vi "Inc_Dec_Builder.vi"(8 "error in (no error)":errorcluster, 9 "Index_Str_In":string, 10 "Array In":i32[](array[numeric])) -> (0 "error out":errorcluster, 2 "Array":i32[](array[numeric]))   [LabVIEW 2017]
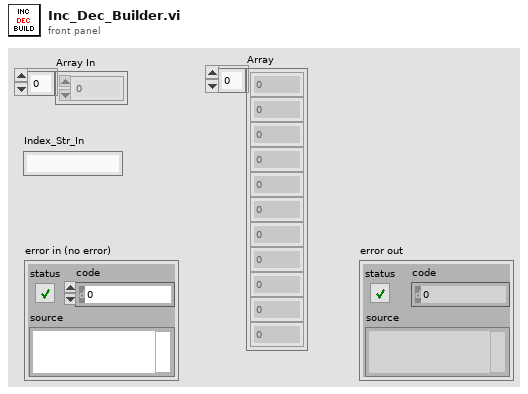
[diagram p1: front panel]
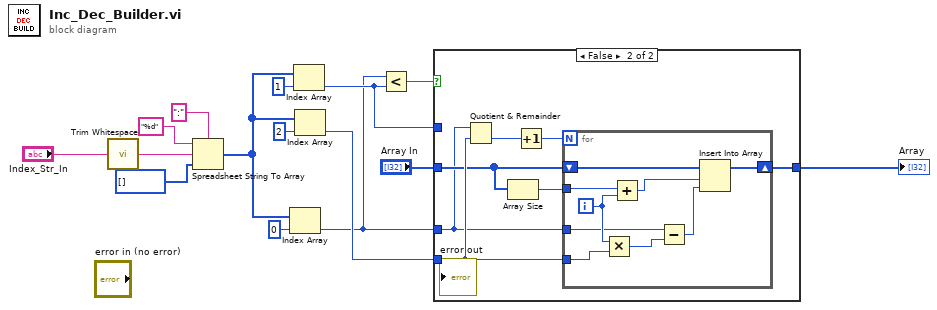
[diagram p0: block diagram]
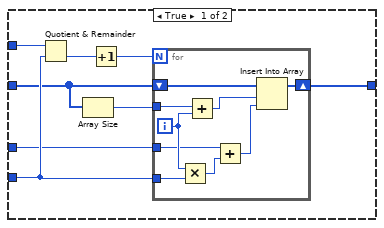
[diagram p2: hidden frame]
diagram:
  n1 = call <vilib>:"Trim Whitespace.vi"("string"="Index_Str_In") -> ("trimmed string"=w13:string)  [unwired: 1 in]
  n2 = Spreadsheet String To Array(delimiter (Tab)=":", format string="%d", spreadsheet string=w13, array type (2D Dbl)=i32[] []) -> (array=w6:i32[])
  n3 = Index Array(array=w6, index=0) -> (element=w1:i32)
  n4 = Index Array(array=w6, index=1) -> (element=w4:i32)
  n5 = Index Array(array=w6, index=2) -> (element=w5:i32)
  n6 = Less?(x=w1, y=w4) -> (x < y?=w8:bool)
  n7 = case shown="False" w8 {
    tunnel: w5 -> [w21 w38]
    tunnel: w4 -> [w23 _]
    tunnel: "Array In" -> [w18 w35]
    tunnel: [w20 w37] -> w2
    tunnel: w1 -> [w16 w33]
    frame True {
      n8 = Quotient & Remainder(x=w23, y=w21) -> (floor(x/y)=w22:i32)  [unwired: 1 out]
      n9 = Array Size(array=w18) -> (size(s)=w17:i32)
      n10 = Increment(x=w22) -> (x+1=w19:i32)
      n11 = for {
        N: w19 -> [_]
        tunnel: w21 -> [w30]
        shift-right: [w31] -> w20
        shift-left: w18 -> [w32]
        tunnel: w17 -> [w29]
        tunnel: w16 -> [w25]
        i -> [w28]
        n12 = Multiply(x=w28, y=w30) -> (x*y=w26:i32)
        n13 = Add(x=w29, y=w28) -> (x+y=w27:i32)
        n14 = Add(x=w25, y=w26) -> (x+y=w24:i32)
        n15 = Insert Into Array(array=w32, index=w27, new element=w24) -> (w31:i32[])
      }
    }
    frame False {
      n16 = Quotient & Remainder(x=w33, y=w38) -> (floor(x/y)=w39:i32)  [unwired: 1 out]
      n17 = Array Size(array=w35) -> (size(s)=w34:i32)
      n18 = Increment(x=w39) -> (x+1=w36:i32)
      n19 = for {
        N: w36 -> [_]
        tunnel: w38 -> [w46]
        shift-right: [w47] -> w37
        shift-left: w35 -> [w48]
        tunnel: w34 -> [w45]
        tunnel: w33 -> [w42]
        i -> [w44]
        n20 = Multiply(x=w44, y=w46) -> (x*y=w41:i32)
        n21 = Add(x=w45, y=w44) -> (x+y=w43:i32)
        n22 = Subtract(x=w42, y=w41) -> (x-y=w40:i32)
        n23 = Insert Into Array(array=w48, index=w43, new element=w40) -> (w47:i32[])
      }
    }
  }
  "Array" <- w2
